vi "APS load amc program.vi"(7 "Password":i32, 8 "error in (no error)":errorcluster caption="错误输入（无错误）", 9 "pFile":string, 10 "TaskNum":i32, 11 "Board_ID":i32) -> (0 "error out":errorcluster caption="错误输出", 3 "function return":i32)   [LabVIEW 2011, in "APS168.lvlib"]
doc: "I32 FNTYPE APS_load_amc_program( I32 Board_ID, I32 TaskNum, const char *pFile, I32 Password);"
uses:
  APS168.lvlib
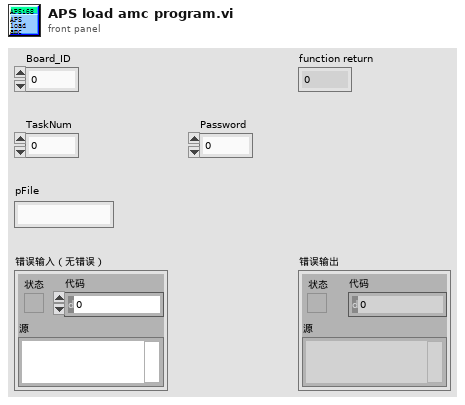
[diagram p1: front panel]
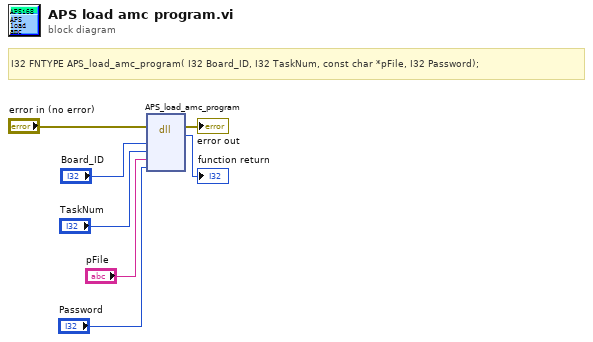
[diagram p0: block diagram]
diagram:
  # "I32 FNTYPE APS_load_amc_program( I32 Board_ID, I32 TaskNum, const char *pFile, I32 Password);"
  n1 = dll-call lib="PTH1Labs E软件ADLINK 204CAPS_1_7_1_LIB line 连续运动204APS168.*" fn="APS_load_amc_program"(error in="error in (no error)", "Board_ID"="Board_ID", "TaskNum"="TaskNum", "pFile"="pFile", "Password"="Password") -> (error out=→"error out":errorcluster, →"function return":i32)  [unwired: 6 in, 1 out]
